vi "Check Status (No Object) - Microwave Amplifier.vi"(8 "error in (no error)":errorcluster, 11 "Cluster In":T1 {"Mode" items=["SLEEP", "WARM-UP", "STANDBY", "OPERATE", "FAULT"]}) -> (0 "error out":errorcluster, 1 "Status":string, 2 "Ready?":bool, 3 "Cluster Out":T1 {"Mode" items=["SLEEP", "WARM-UP", "STANDBY", "OPERATE", "FAULT"]})   [LabVIEW 2012]
doc: "(Dynamic) Check if the instrument is powered on and update its member fields with the instrument's current status. Optionally return a text status message."
uses:
  Global/GPIB Numbers.vi
  Microwave Amp/MicrowaveAmplifier.lvlib
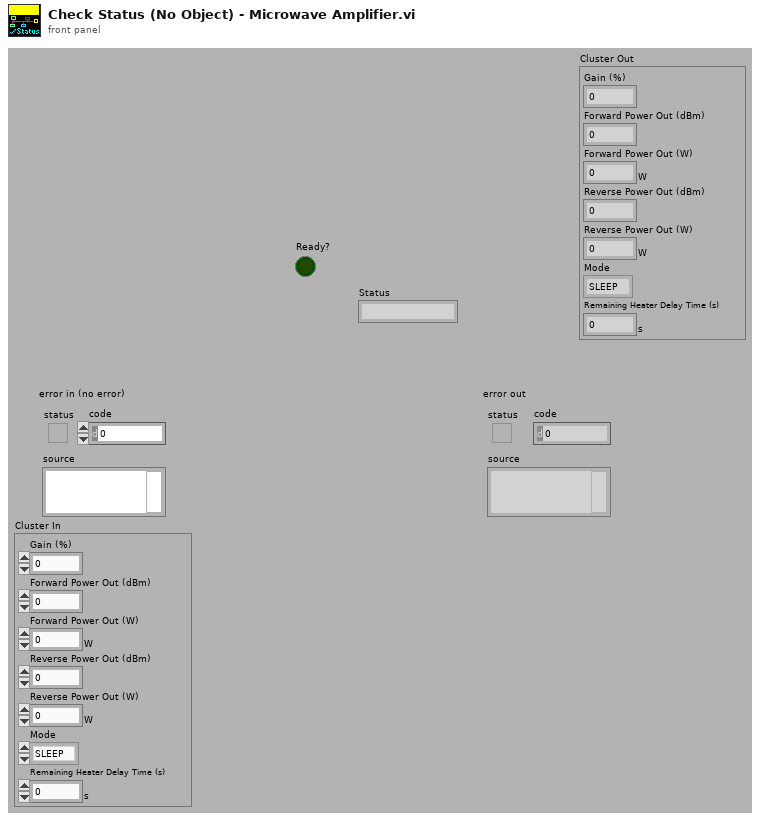
[diagram p1: front panel]
types:
  T1 = cluster{"Gain (%)":dbl, "Forward Power Out (dBm)":dbl, "Forward Power Out (W)":dbl[unit], "Reverse Power Out (dBm)":dbl, "Reverse Power Out (W)":dbl[unit], "Mode":u16, "Remaining Heater Delay Time (s)":dbl[unit]}
  T2 = typedef "GPIB Type Def.ctl" = cluster{"Name":string, "bus":dbl, "GPIB":dbl, "GPIB as string":string, "byte":i32, "VISA Resource Name":refnum<visa-resource-name>}
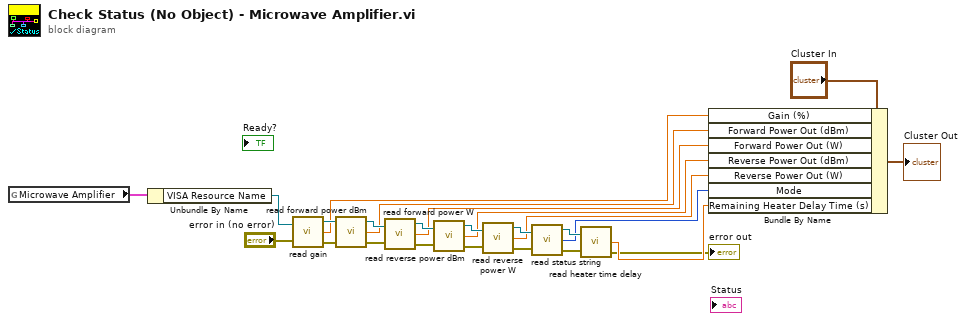
[diagram p0: block diagram]
diagram:
  n1 = global read "GPIB Numbers.vi" "Microwave Amplifier"() -> (w2:T2)
  n2 = Unbundle By Name(w2) -> ("VISA Resource Name"=w1:refnum<visa-resource-name>)
  n3 = call "read gain.vi"("VISA resource name"=w1, "error in (no error)"="error in (no error)") -> ("VISA resource name out"=w19:refnum<visa-resource-name>, "Gain (%)"=w13:dbl, "error out"=w25:errorcluster)
  n4 = call "read forward power dBm.vi"("error in (no error)"=w25, "VISA resource name"=w19) -> ("error out"=w24:errorcluster, "forward power (dBm)"=w12:dbl, "VISA resource name out"=w18:refnum<visa-resource-name>)  [unwired: 1 in]
  n5 = call "read forward power W.vi"("VISA resource name"=w18, "error in (no error)"=w24) -> ("VISA resource name out"=w17:refnum<visa-resource-name>, "foward power (W)"=w11:dbl[unit], "error out"=w23:errorcluster)
  n6 = call "read reverse power dBm.vi"("VISA resource name"=w17, "error in (no error)"=w23) -> ("VISA resource name out"=w16:refnum<visa-resource-name>, "reverse power (dBm)"=w10:dbl, "error out"=w22:errorcluster)
  n7 = call "read reverse power W.vi"("VISA resource name"=w16, "error in (no error)"=w22) -> ("VISA resource name out"=w15:refnum<visa-resource-name>, "Reverse Power (W)"=w9:dbl[unit], "error out"=w21:errorcluster)
  n8 = call "read status string.vi"("VISA resource name"=w15, "error in (no error)"=w21) -> ("VISA resource name out"=w14:refnum<visa-resource-name>, "Mode"=w8:u16, "error out"=w20:errorcluster)
  n9 = call "read heater time delay.vi"("VISA resource name"=w14, "error in (no error)"=w20) -> ("Heater delay time (s)"=w7:dbl[unit], "error out"=→"error out":errorcluster)  [unwired: 1 out]
  n10 = Bundle By Name(cluster="Cluster In", "Gain (%)"=w13, "Forward Power Out (dBm)"=w12, "Forward Power Out (W)"=w11, "Reverse Power Out (dBm)"=w10, "Reverse Power Out (W)"=w9, "Mode"=w8, "Remaining Heater Delay Time (s)"=w7) -> (→"Cluster Out":T1)
